vi "Read_action.vi"(8 "error in (no error)":errorcluster, 11 "MyAppConfig in":refnum<class "MyAppConfig.lvclass">) -> (0 "error out":errorcluster, 2 "All items found?":bool, 3 "MyAppConfig out":refnum<class "MyAppConfig.lvclass">)   [LabVIEW 2012, in "MyApp.lvlib" / "MyAppConfig.lvclass"]
uses:
  MyAppConfig.lvclass
  HGF_LVC/HGF_ApplicationBaseClasses/HGF_Configuration/HGF_Configuration.lvclass
  MyAppConfig.lvclass/MyAppConfig.ctl
  <vilib>/Utility/config.llb/Read Key (String).vi
  <vilib>/Utility/config.llb/Read Key (I32).vi
  <vilib>/Utility/config.llb/NI_LVConfig.lvlib
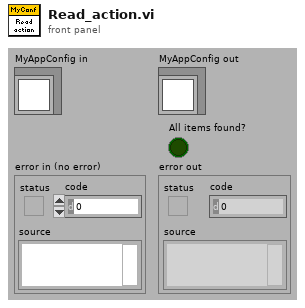
[diagram p1: front panel]
types:
  T1 = typedef "NI_LVConfig.lvlib/Config Data RefNum.ctl" = refnum<k1>
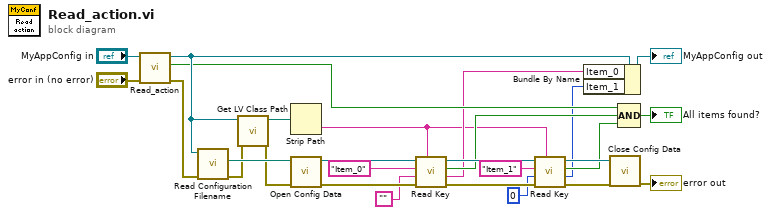
[diagram p0: block diagram]
diagram:
  n1 = call-parent "Read_action.vi"("error in (no error)"="error in (no error)", "HGF_Configuration in"="MyAppConfig in") -> ("error out"=w25:errorcluster, "All items found?"=w8:bool, "HGF_Configuration out"=w21:refnum<class "MyAppConfig.lvclass">)  [unwired: 7 in]
  n2 = call "Read Configuration Filename.vi"("error in (no error)"=w25, "HGF_Configuration in"=w21) -> ("error out"=w19:errorcluster, "Configuration Filename"=w24:path)  [unwired: 7 in, 1 out]
  n3 = call <vilib>:"Get LV Class Path.vi"("error in (no error)"=w19, "object"=w21) -> ("error out"=w18:errorcluster, "class path"=w20:path)  [unwired: 8 in]
  n4 = Strip Path(path=w20) -> (name=w1:string)  [unwired: 1 out]
  n5 = call <vilib>:"Open Config Data.vi"("error in (no error)"=w18, "configuration file path"=w24) -> ("error out"=w22:errorcluster, "refnum"=w23:T1)  [unwired: 7 in, 1 out]
  n6 = call-poly <vilib>:"Read Key.vi"("section"=w1, "error in (no error)"=w22, "default value"="", "key"="Item_0", "refnum"=w23) -> ("error out"=w14:errorcluster, "value"=w3:string, "found?"=w7:bool, "refnum out"=w15:T1)  [unwired: 3 in]
  n7 = call-poly <vilib>:"Read Key.vi"("section"=w1, "error in (no error)"=w14, "default value"=0, "key"="Item_1", "refnum"=w15) -> ("error out"=w11:errorcluster, "value"=w2:i32, "found?"=w6:bool, "refnum out"=w10:T1)  [unwired: 3 in]
  n8 = Bundle By Name(cluster=w21, "Item_0"=w3, "Item_1"=w2) -> (→"MyAppConfig out":refnum<class "MyAppConfig.lvclass">)
  n9 = call <vilib>:"Close Config Data.vi"("error in (no error)"=w11, "refnum"=w10) -> ("error out"=→"error out":errorcluster)  [unwired: 8 in, 1 out]
  n10 = Compound Arithmetic op=AND(w8, w7, w6) -> (→"All items found?":bool)
